vi "RunTimeMissing Dialog.vi"(5 "error in":errorcluster) -> (19 "error out":errorcluster)   [LabVIEW 2020, in "DP_WebView.lvclass"]
uses:
  DP_WebView.lvclass
  <vilib>/Platform/browser.llb/Open URL in Default Browser (string).vi
panel:
  in  "Close":bool
  in  "Exit":bool
  in  "Download":bool
  out "Link":string
  # "Webview2 Run-Time engine missing"
  # "This application required the Webview2 Run-Time engine,\nwhich couldn't be found.\n\nPlease install this and restart the application.\n\nDownload it from here:"
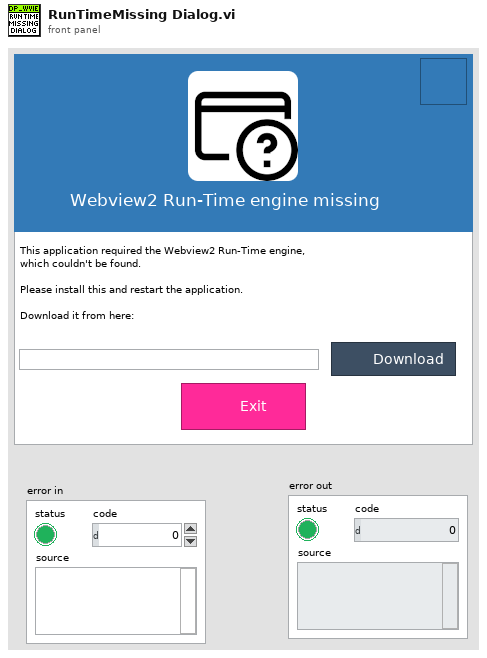
[diagram p1: front panel]
types:
  T1 = typedef "LVRectTypeDef.ctl" = cluster{"Left":i16, "Top":i16, "Right":i16, "Bottom":i16}
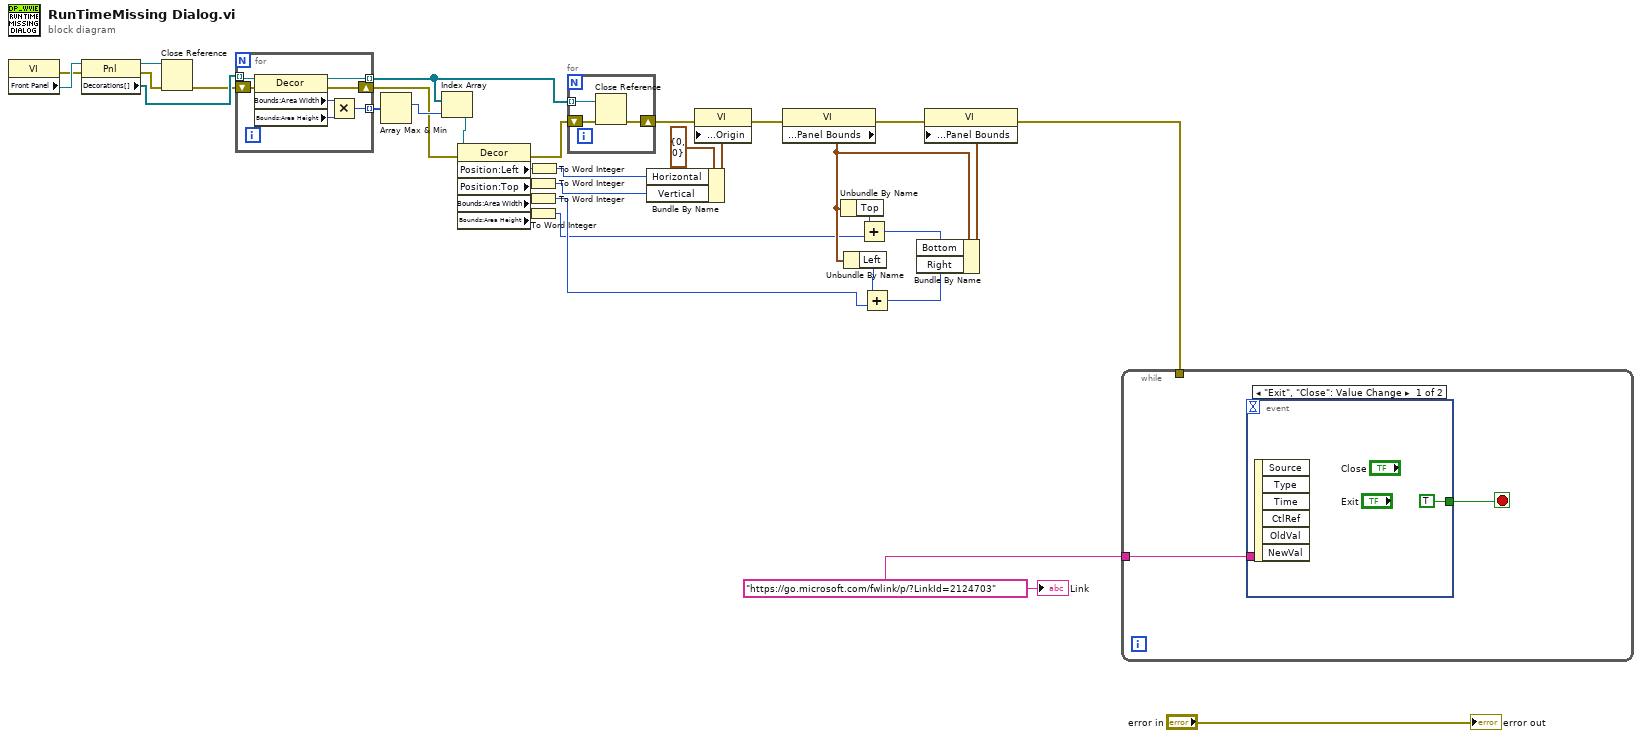
[diagram p0: block diagram]
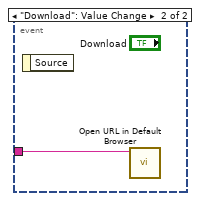
[diagram p2: hidden frame]
diagram:
  w34 = "https://go.microsoft.com/fwlink/p/?LinkId=2124703" ("Link")
  n1 = property on="Property Node" class="VI"() -> (error out=w28:errorcluster, "Front Panel"=w30:refnum<vi>)  [unwired: 2 in, 1 out]
  n2 = property on="Property Node" class="Pnl"(reference=w30, error in=w28) -> (reference out=w27:refnum<vi>, error out=w29:errorcluster, "Decorations[]"=w32:refnum<vi>[])
  n3 = Close Reference(reference=w27, error in (no error)=w29) -> (error out=w31:errorcluster)
  n4 = for {
    tunnel: w32 -> [w41] mode=indexing
    tunnel: [w38] -> w15 mode=indexing
    shift-right: [w36] -> w11
    shift-left: w31 -> [w37]
    tunnel: [w35] -> w13 mode=indexing
    n5 = property class="Decor"(reference=w41, error in=w37) -> (reference out=w35:refnum<vi>, error out=w36:errorcluster, "Bounds:Area Width"=w40:u32, "Bounds:Area Height"=w39:u32)
    n6 = Multiply(x=w40, y=w39) -> (x*y=w38:u32)
  }
  n7 = Array Max & Min(array=w15) -> (max index (indices)=w14:i32)  [unwired: 3 out]
  n8 = Index Array(array=w13, index=w14) -> (element=w12:refnum<vi>)
  n9 = property class="Decor"(reference=w12, error in=w11) -> (error out=w10:errorcluster, "Position:Left"=w18:i32, "Position:Top"=w19:i32, "Bounds:Area Width"=w24:u32, "Bounds:Area Height"=w22:u32)  [unwired: 1 out]
  n10 = To Word Integer(number=w19) -> (16bit integer=w3:i16)
  n11 = To Word Integer(number=w24) -> (16bit integer=w6:i16)
  n12 = To Word Integer(number=w22) -> (16bit integer=w5:i16)
  n13 = To Word Integer(number=w18) -> (16bit integer=w4:i16)
  n14 = for {
    tunnel: w13 -> [w44] mode=indexing
    shift-right: [w42] -> w9
    shift-left: w10 -> [w43]
    n15 = Close Reference(reference=w44, error in (no error)=w43) -> (error out=w42:errorcluster)
  }
  n16 = Bundle By Name(cluster=cluster{"Horizontal":i16, "Vertical":i16} {"Horizontal"=0, "Vertical"=0} ("Front Panel Window:Origin"), "Horizontal"=w4, "Vertical"=w3) -> (w16:cluster{"Horizontal":i16, "Vertical":i16})
  n17 = property on="Property Node" class="VI"(error in=w9, "Front Panel Window:Origin"=w16) -> (error out=w8:errorcluster)  [unwired: 1 in, 1 out]
  n18 = property on="Property Node" class="VI"(error in=w8) -> (error out=w7:errorcluster, "Front Panel Window:Panel Bounds"=w20:T1)  [unwired: 1 in, 1 out]
  n19 = Unbundle By Name(w20) -> ("Top"=w21:i16)
  n20 = Unbundle By Name(w20) -> ("Left"=w23:i16)
  n21 = Add(x=w21, y=w5) -> (x+y=w2:i16)
  n22 = Add(x=w23, y=w6) -> (x+y=w1:i16)
  n23 = Bundle By Name(cluster=w20, "Bottom"=w2, "Right"=w1) -> (w25:T1)
  n24 = property on="Property Node" class="VI"(error in=w7, "Front Panel Window:Panel Bounds"=w25) -> (error out=w26:errorcluster)  [unwired: 1 in, 1 out]
  n25 = while {
    tunnel: w34 -> [w45]
    tunnel: w26 -> [_]
    stop <- w46 stop-if-true
    n26 = event shown="[0] \"Exit\", \"Close\": Value Change" {
      selector: _ -> [_ _]
      dyn-events: _ -> [_ _]
      timeout: _ -> [_ _]
      tunnel: [TRUE _] -> w46
      tunnel: w45 -> [_ w48]
      event "Exit", "Close": Value Change {
        n27 = event-data() -> ()  [unwired: 1 in, 6 out]
      }
      event "Download": Value Change {
        n28 = event-data() -> ()  [unwired: 1 in, 1 out]
        n29 = call-poly <vilib>:"Open URL in Default Browser.vi"("URL"=w48) -> ()  [unwired: 5 in, 2 out]
      }
    }
  }
  "Link" <- w34
  "error out" <- "error in"
